vi "get data frame.vi"(11 "字符串":string) -> (1 "标记位":bool, 2 "匹配+剩余字符串":string, 3 "匹配之前的子字符串":string)   [LabVIEW 2016, in "EXO2-Sonde.lvlib"]
uses:
  EXO2-Sonde.lvlib
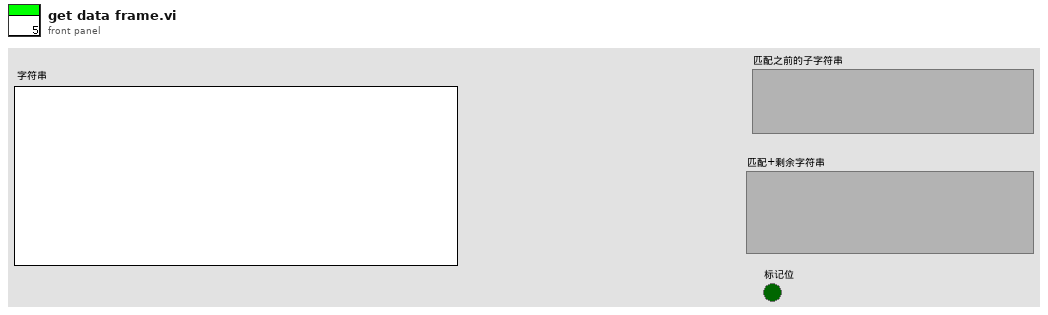
[diagram p1: front panel]
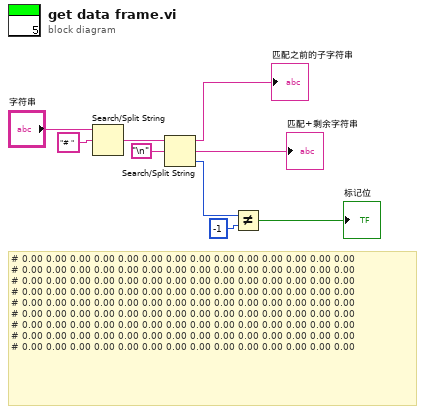
[diagram p0: block diagram]
diagram:
  # "# 0.00 0.00 0.00 0.00 0.00 0.00 0.00 0.00 0.00 0.00 0.00 0.00 0.00 0.00 \n# 0.00 0.00 0.00 0.00 0.00 0.00 0.00 0.00 0.00 0.00 0.00 0.00 0.00 0.00 \n# 0.00 0.00 0.00 0.00 0.00 0.00 0.00 0.00 0.00 0.00 0.00 0.00 0.00 0.00 \n# 0.00 0.00 0.00 0.00 0.00 0.00 0.00 0.00 0.00 0.00 0.00 0.00 0.00 0.00 \n# 0.00 0.00 0.00 0.00 0.00 0.00 0.00 0.00 0.00 0.00 0.00 0.00 0.00 0.00 \n# 0.00 0.00 0.00 0.00 0.00 0.00 0.00 0.00 0.00 0.00 0.00 0.00 0.00 0.00 \n# 0.00 0.00 0.00 0.00 0.00 0.00 0.00 0.00 0.00 0.00 0.00 0.00 0.00 0.00 \n# 0.00 0.00 0.00 0.00 0.00 0.00 0.00 0.00 0.00 0.00 0.00 0.00 0.00 0.00 \n# 0.00 0.00 0.00 0.00 0.00 0.00 0.00 0.00 0.00 0.00 0.00 0.00 0.00 0.00"
  n1 = Search/Split String(string="字符串", search string/char (-)="# " ("搜索字符串/字符(-)")) -> (match + rest of string=w7:string)  [unwired: 1 in, 2 out]
  n2 = Search/Split String(string=w7, search string/char (-)="\n") -> (substring before match=→"匹配之前的子字符串":string, match + rest of string=→"匹配+剩余字符串":string, offset of match=w4:i32)  [unwired: 1 in]
  n3 = Not Equal?(x=w4, y=-1) -> (x != y?=→"标记位":bool)
